vi "Configure Acquisition Type.vi"(6 "Average Number (2)":i32=2, 8 "error in (no error)":errorcluster, 9 "Sample Mode (0: Real Time)":u16(ring) items=["Real Time"], 10 "Acquisition Type (0: Normal)":u16(ring) items=["Normal", "Peak Detect", "Average"], 11 "VISA resource name":refnum<visa-resource-name>) -> (0 "error out":errorcluster, 3 "VISA resource name out":refnum<visa-resource-name>)   [LabVIEW 2010, in "Agilent DSO1000 Series.lvlib"]
doc: "Configures how the oscilloscope accquires the data and fills the waveform record."
uses:
  <instrlib>/Agilent DSO1000 Series/Agilent DSO1000 Series.lvlib
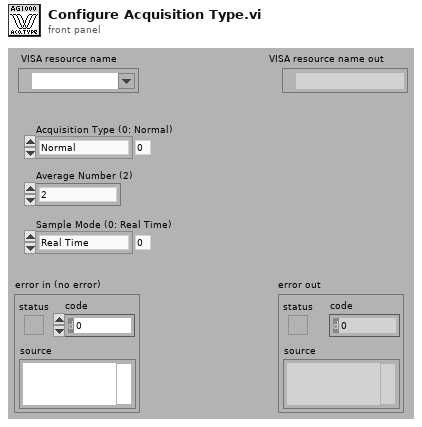
[diagram p1: front panel]
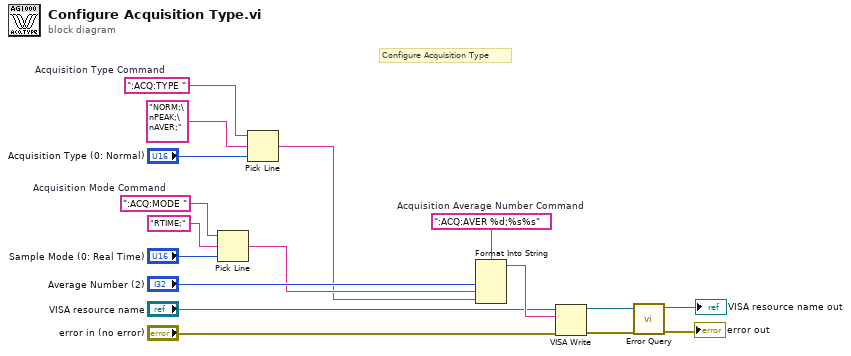
[diagram p0: block diagram]
diagram:
  w10 = ":ACQ:TYPE "  # Acquisition Type Command
  w13 = ":ACQ:AVER %d;%s%s"  # Acquisition Average Number Command
  w16 = ":ACQ:MODE "  # Acquisition Mode Command
  # "Configure Acquisition Type"
  n1 = Pick Line(string ("")=w16, multi-line string="RTIME;" ("string (\"\")"), line index="Sample Mode (0: Real Time)") -> (output string=w6:string)
  n2 = Pick Line(string ("")=w10, multi-line string="NORM;\nPEAK;\nAVER;", line index="Acquisition Type (0: Normal)") -> (output string=w5:string)
  n3 = Format Into String(format string=w13, "Average Number (2)", w6, w5) -> (resulting string=w12:string)  [unwired: 2 in, 1 out]
  n4 = VISA Write(VISA resource name="VISA resource name", write buffer=w12, error in (no error)="error in (no error)") -> (VISA resource name out=w2:refnum<visa-resource-name>, error out=w1:errorcluster)  [unwired: 1 out]
  n5 = call <instrlib>:"Error Query.vi"("error in (no error)"=w1, "VISA resource name"=w2) -> ("error out"=→"error out":errorcluster, "VISA resource name out"=→"VISA resource name out":refnum<visa-resource-name>)  [unwired: 6 in, 2 out]
